vi "test_harness_Hyst_op_fxp_16_5.vi"() -> ()   [LabVIEW 2019, in "Sat_Hyst_TestCase.lvclass"]
uses:
  Sat_Hyst_TestCase.lvclass
  C:/Program Files (x86)/National Instruments/LabVIEW 2019/vi.lib/addons/_JKI Toolkits/VI Tester/TestCase.llb/TestCase.lvclass
  hyst_sat_fxp_16_5_weights.ctl
  <vilib>/rvi/DesktopExecutionNode/Execution/niFpgaDEN_Execute.vi
  <vilib>/rvi/DesktopExecutionNode/DesktopExecutionNode.xnode
  <vilib>/Wiresmith Technology/VITAC (VI Tester Advanced Comparisons)/VITAC.lvlib
panel:
  out "Cluster":T1
  out "U_nom":dbl[](array[numeric])
  out "N_traj":i32
  out "sat_inv(unom)":dbl[](array[numeric])
  in  "Path":path=path "C:/Users/arnold/Documents/matlab/afm_mpc_journal/unit_tests/labview/hyst_sat_data.csv"
  out "y_out_mem":fxp<+/-,16,5>[](array[numeric])
  out "S_of_ik (expected)":sgl[](array[numeric])
  in  "error in (no error)":errorcluster
  out "error out":errorcluster
  out "TestCase out":refnum<class "Sat_Hyst_TestCase.lvclass">
  in  "TestCase in":refnum<class "Sat_Hyst_TestCase.lvclass">
  out "H_of_uk":fxp<+/-,32,10>[](array[numeric])
  out "hinv(satinv)":dbl[](array[numeric])
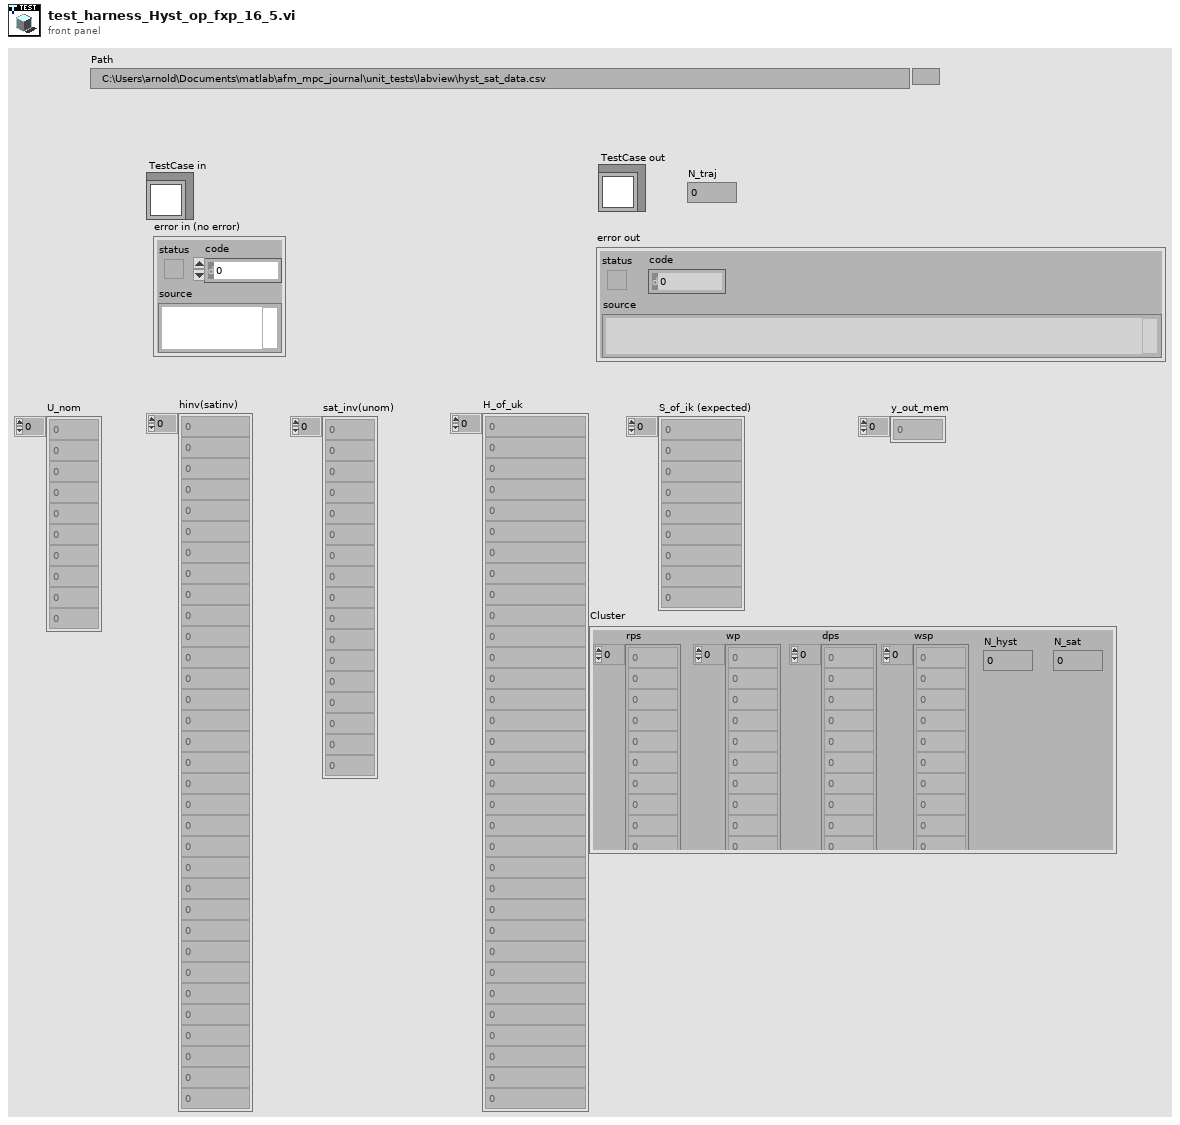
[diagram p1: front panel]
types:
  T1 = typedef "hyst_sat_fxp_16_5_weights.ctl" = cluster{"rps":dbl[], "wp":dbl[], "dps":dbl[], "wsp":dbl[], "N_hyst":i32, "N_sat":i32}
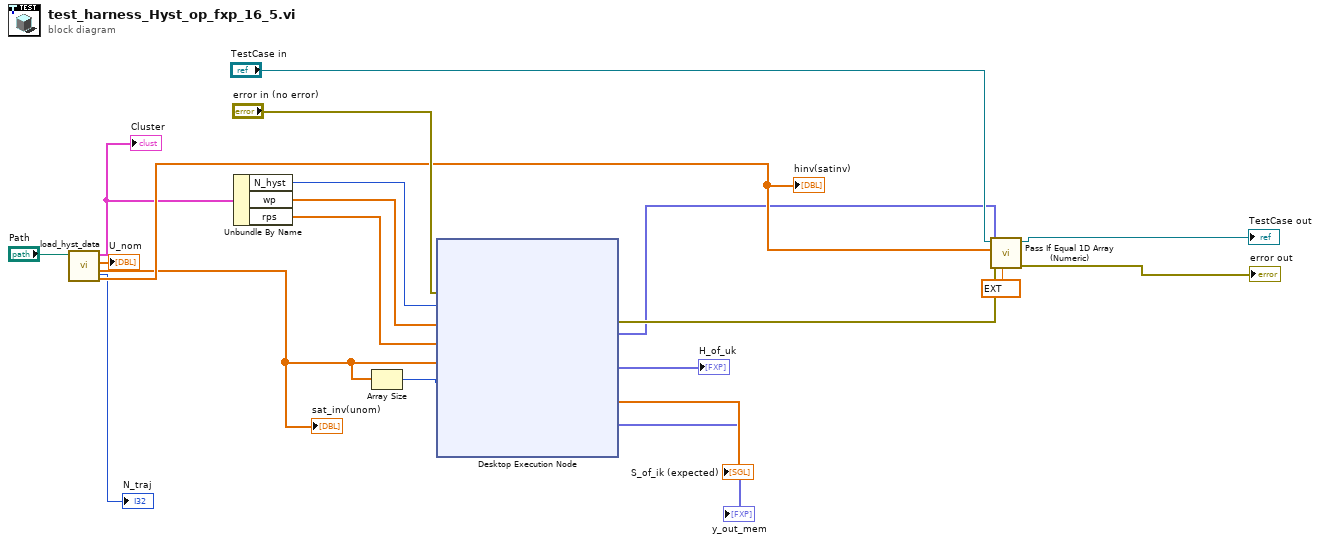
[diagram p0: block diagram]
diagram:
  n1 = call "load_hyst_data.vi"("Path"="Path") -> ("h_inv(u_satinv)"=w13:dbl[], "sat_inv(u_nom)"=w12:dbl[], "U_nom"=→"U_nom":dbl[], "Cluster"=w5:T1, "N_traj"=→"N_traj":i32)  [unwired: 6 in]
  "hinv(satinv)" <- w13
  "sat_inv(unom)" <- w12
  "Cluster" <- w5
  n2 = Unbundle By Name(w5) -> ("N_hyst"=w4:i32, "wp"=w2:dbl[], "rps"=w1:dbl[])
  n3 = Array Size(array=w12) -> (size(s)=w11:i32)
  n4 = xnode "Desktop Execution Node"("Error In"="error in (no error)", "N_hyst"=w4, "w_s"=w2, "r_s"=w1, "uk"=w12, "numIter"=w11) -> ("Error Out"=w16:errorcluster, "H_of_uk"=w10:fxp<+/-,32,10>[], "S_of_ik (expected)"=→"S_of_ik (expected)":sgl[], "y_out_mem"=→"y_out_mem":fxp<+/-,16,5>[])
  "H_of_uk" <- w10
  n5 = call <vilib>:"Pass If Equal 1D Array (Numeric).vi"("delta (optional)"=ext 0.0001, "error in (no error)"=w16, "actual"=w10, "expected"=w13, "TestCase in"="TestCase in") -> ("error out"=→"error out":errorcluster, "TestCase out"=→"TestCase out":refnum<class "Sat_Hyst_TestCase.lvclass">)  [unwired: 5 in]
